vi "crossing counter panel.vi"() -> ()   [LabVIEW 2017]
uses:
  control panel globals.vi
panel:
  out "rms amplitude":dbl
  out "error out":errorcluster
  in  "stop counting":bool
  in  "start counting":bool
  in  "crossings to count":u32
  out "elapsed time":dbl format="%.3f"
  out "number of full crossings":dbl format="%.2f"
  # "s"
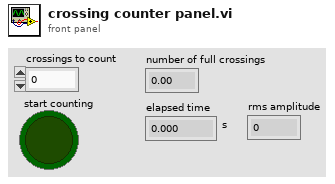
[diagram p1: front panel]
types:
  T1 = typedef "queue cluster.ctl" = cluster{"voltage":T2, "coil":T2, "mag":refnum<queue>, "accel":T2, "crossing":T2, "orbit fit":refnum<queue>, "pulse":T2, "mag0":T2, "fitLocation":refnum<queue>}
  T2 = typedef "reading queue.ctl" = refnum<queue>
  T3 = typedef "reading.ctl" = cluster{"reading type":T4, "time":fxp<+,48,48>, "x":sgl, "y":sgl, "z":sgl, "XSUM":u8}
  T4 = typedef "readingType.ctl" = enum8{"SYNC", "DETVAL", "COILI", "MAGVEC", "ACCVEC", "CROSSING", "MAGVEC0", "MAGVEC1", "MAGVEC2", "MAGVEC3", "MAGVEC4", "MAGVEC5", "MAGVEC6", "MAGVEC7"}
  T5 = typedef "orbit parameters with crossing info.ctl" = cluster{"a":dbl, "b":dbl, "theta_axis":dbl, "dPhi":dbl, "BrV":dbl, "bob tilt":dbl, "phi0":dbl, "phi_dot":dbl, "x0":dbl, "y0":dbl, "z0":dbl, "mid crossing time":dbl, "most recent crossing number":dbl, "most recent crossing slope":dbl, "most recent crossing period":dbl}
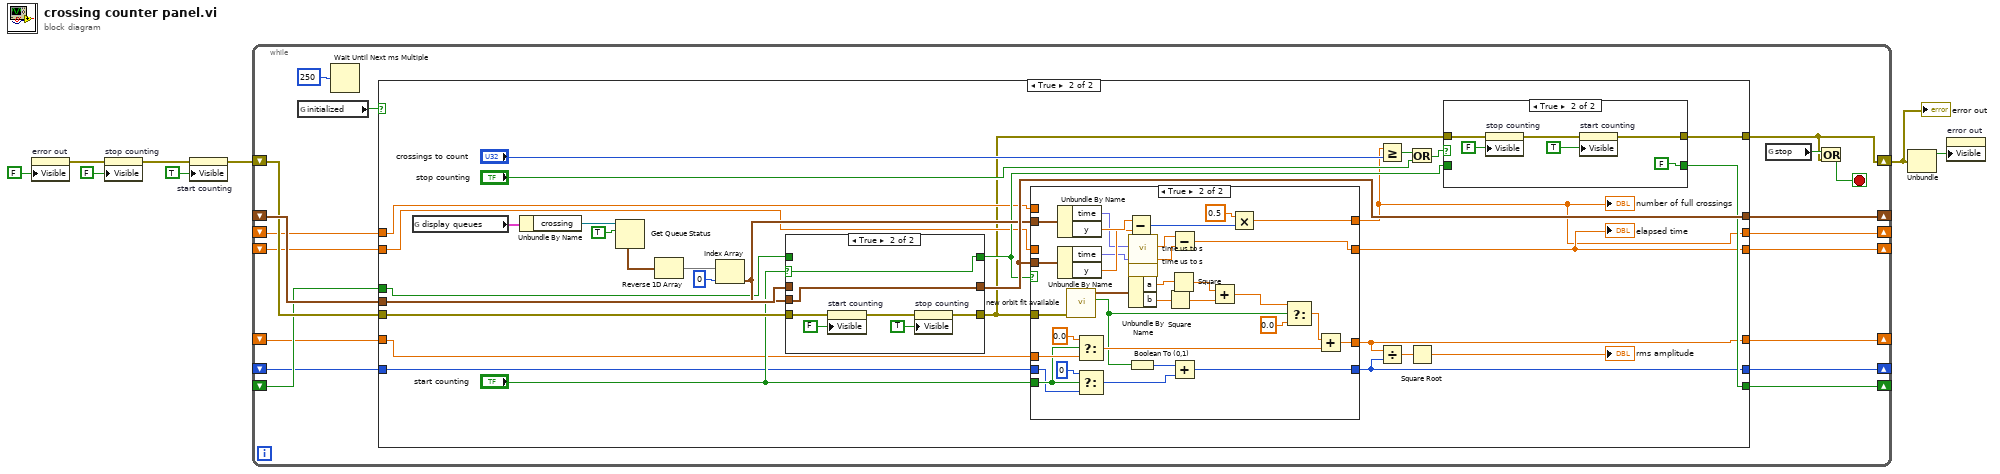
[diagram p0: block diagram]
diagram:
  n1 = property on="error out" class="Clust (strict)"("Visible"=FALSE) -> (error out=w4:errorcluster)  [unwired: 2 in, 1 out]
  n2 = property on="stop counting" class="Bool"(error in=w4, "Visible"=FALSE) -> (error out=w6:errorcluster)  [unwired: 1 in, 1 out]
  n3 = property on="start counting" class="Bool"(error in=w6, "Visible"=TRUE) -> (error out=w5:errorcluster)  [unwired: 1 in, 1 out]
  n4 = while {
    shift-right: [w24] -> _
    shift-left: _ -> [w26]
    shift-right: [w14] -> w2
    shift-left: w5 -> [w25]
    shift-right: [w23] -> _
    shift-left: _ -> [w22]
    shift-right: [w21] -> _
    shift-left: _ -> [w19]
    shift-right: [w20] -> _
    shift-left: _ -> [w18]
    shift-right: [w12] -> _
    shift-left: _ -> [w10]
    shift-right: [w11] -> _
    shift-left: _ -> [w9]
    stop <- w13 stop-if-true
    n5 = global read "control panel globals.vi" "initialized"() -> (w17:bool)
    n6 = Wait Until Next ms Multiple(millisecond multiple=u32 250) -> ()  [unwired: 1 out]
    n7 = case shown="True" w17 {
      tunnel: w26 -> [w30 w57]
      tunnel: w25 -> [w32 w56]
      tunnel: [w30 w55] -> w24
      tunnel: [w31 w48] -> w23
      tunnel: w22 -> [w31 w47]
      tunnel: [w32 w46] -> w14
      tunnel: [w33 w45] -> w21
      tunnel: [w29 w44] -> w20
      tunnel: w19 -> [w33 w43]
      tunnel: w18 -> [w29 w42]
      tunnel: [w28 w39] -> w12
      tunnel: [w27 w38] -> w11
      tunnel: w10 -> [w28 w35]
      tunnel: w9 -> [w27 w34]
      frame False {
      }
      frame True {
        n8 = global read "control panel globals.vi" "display queues"() -> (w60:T1)
        n9 = Unbundle By Name(w60) -> ("crossing"=w61:T2)
        n10 = Get Queue Status(queue=w61, return elements? (F)=TRUE) -> (elements=w62:T3[])  [unwired: 1 in, 7 out]
        n11 = Reverse 1D Array(array=w62) -> (reversed array=w63:T3[])
        n12 = Index Array(array=w63, index=0) -> (element=w54:T3)
        n13 = case shown="True" "start counting" {
          selector: "start counting" -> [_ w111]
          tunnel: [w110 w112] -> w55
          tunnel: w54 -> [_ w112]
          tunnel: w57 -> [w110 _]
          tunnel: w56 -> [w108 w115]
          tunnel: [w108 w113] -> w41
          tunnel: [w109 w111] -> w49
          tunnel: w47 -> [w109 _]
          frame False {
          }
          frame True {
            n14 = property on="start counting" class="Bool"(error in=w115, "Visible"=FALSE) -> (error out=w114:errorcluster)  [unwired: 1 in, 1 out]
            n15 = property on="stop counting" class="Bool"(error in=w114, "Visible"=TRUE) -> (error out=w113:errorcluster)  [unwired: 1 in, 1 out]
          }
        }
        n16 = case shown="True" w49 {
          tunnel: w55 -> [_ w106]
          tunnel: w54 -> [_ w107]
          tunnel: [w75 w105] -> w45
          tunnel: [w74 w101] -> w44
          tunnel: w43 -> [w75 _]
          tunnel: w42 -> [w74 _]
          tunnel: w41 -> [_ w95]
          tunnel: "start counting" -> [_ w81]
          tunnel: [w72 w76] -> w38
          tunnel: [w73 w86] -> w39
          tunnel: w35 -> [w73 w85]
          tunnel: w34 -> [w72 w80]
          frame False {
          }
          frame True {
            n17 = Unbundle By Name(w107) -> ("time"=w99:fxp<+,48,48>, "y"=w104:sgl)
            n18 = Unbundle By Name(w106) -> ("time"=w97:fxp<+,48,48>, "y"=w103:sgl)
            n19 = call "new orbit fit available.vi"("error in (no error)"=w95) -> ("new fit available"=w78:bool, "orbit fit"=w94:T5)  [unwired: 8 in, 1 out]
            n20 = Select(t=0.0, s=w81, f=w85) -> (s? t:f=w84:dbl)
            n21 = Select(t=0, s=w81, f=w80) -> (s? t:f=w79:i32)
            n22 = Subtract(x=w104, y=w103) -> (x-y=w102:i32)
            n23 = Boolean To (0,1)(Boolean=w78) -> (0, 1=w77:i16)
            n24 = call "time us to s.vi"("time (us)"=w99) -> ("time (s)"=w98:dbl)  [unwired: 10 in]
            n25 = call "time us to s.vi"("time (us)"=w97) -> ("time (s)"=w96:dbl)  [unwired: 10 in]
            n26 = Unbundle By Name(w94) -> ("a"=w93:dbl, "b"=w92:dbl)
            n27 = Square(x=w92) -> (x^2=w90:dbl)
            n28 = Square(x=w93) -> (x^2=w91:dbl)
            n29 = Subtract(x=w98, y=w96) -> (x-y=w105:dbl)
            n30 = Add(x=w77, y=w79) -> (x+y=w76:i32)
            n31 = Add(x=w91, y=w90) -> (x+y=w89:dbl)
            n32 = Multiply(x=0.5, y=w102) -> (x*y=w101:dbl)
            n33 = Select(t=w89, s=w78, f=0.0) -> (s? t:f=w87:dbl)
            n34 = Add(x=w87, y=w84) -> (x+y=w86:dbl)
          }
        }
        "elapsed time" <- w45
        "number of full crossings" <- w44
        n35 = Greater Or Equal?(x=w44, y="crossings to count") -> (x >= y?=w52:bool)
        n36 = Divide(x=w39, y=w38) -> (x/y=w37:dbl)
        n37 = Or(x=w52, y="stop counting") -> (x .or. y?=w50:bool)
        n38 = Square Root(x=w37) -> (sqrt(x)=→"rms amplitude":dbl)
        n39 = case shown="True" w50 {
          tunnel: w41 -> [w64 w68]
          tunnel: [w64 w67] -> w46
          tunnel: w49 -> [w65 _]
          tunnel: [w65 FALSE] -> w48
          frame False {
          }
          frame True {
            n40 = property on="stop counting" class="Bool"(error in=w68, "Visible"=FALSE) -> (error out=w69:errorcluster)  [unwired: 1 in, 1 out]
            n41 = property on="start counting" class="Bool"(error in=w69, "Visible"=TRUE) -> (error out=w67:errorcluster)  [unwired: 1 in, 1 out]
          }
        }
      }
    }
    n42 = global read "control panel globals.vi" "stop"() -> (w15:bool)
    n43 = Or(x=w15, y=w14) -> (x .or. y?=w13:bool)
  }
  "error out" <- w2
  n44 = Unbundle(w2) -> ("status"=w1:bool)  [unwired: 2 out]
  n45 = property on="error out" class="Clust (strict)"("Visible"=w1) -> ()  [unwired: 2 in, 2 out]
